vi "promedio(muchos controles.vi"() -> ()   [LabVIEW 2017]
panel:
  in  "stop":bool
  out "Promedio":dbl
  out "Dato actual":dbl
  # "This Vi will\nshow the mean\nof the last four elements of \na random generator \ndata"
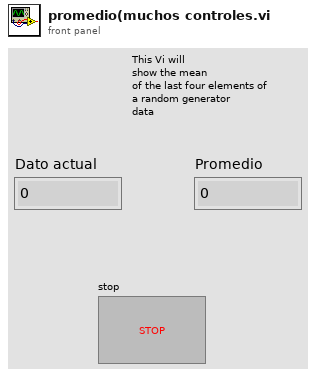
[diagram p1: front panel]
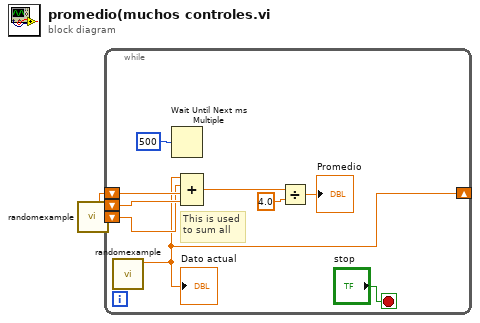
[diagram p0: block diagram]
diagram:
  n1 = call "randomexample.vi"() -> ("Numeric"=w1:dbl)  [unwired: 11 in]
  n2 = while {
    shift-right: [w4] -> _
    shift-left: w1 -> [w10]
    shift-left: w1 -> [w8]
    shift-left: w1 -> [w9]
    stop <- "stop" stop-if-true
    # "This is used\nto sum all"
    n3 = call "randomexample.vi"() -> ("Numeric"=w4:dbl)  [unwired: 11 in]
    "Dato actual" <- w4
    n4 = Wait Until Next ms Multiple(millisecond multiple=u32 500) -> ()  [unwired: 1 out]
    n5 = Compound Arithmetic op=ADD(w4, w8, w10, w9) -> (w6:dbl)
    n6 = Divide(x=w6, y=4.0) -> (x/y=→"Promedio":dbl)
  }
